vi "Decode_Int16.vi"(1 "Little Endian":u8[](array[numeric])) -> (0 "Int16":i16[](array[numeric]))   [LabVIEW 2015, in "navX Library v3.lvlib" / "navX Registry Cache.lvclass"]
uses:
  navX Registry Cache.lvclass
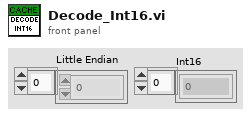
[diagram p1: front panel]
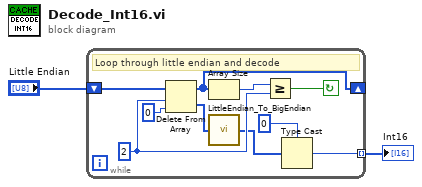
[diagram p0: block diagram]
diagram:
  n1 = while {
    shift-right: [w3] -> _
    shift-left: "Little Endian" -> [w7]
    tunnel: [w5] -> w1 mode=indexing
    stop <- w4 continue-if-true
    w9 = 2 ("length")
    # "Loop through little endian and decode"
    n2 = Delete From Array(array=w7, length=w9, index=0) -> (deleted portion=w8:u8[], array with subset deleted=w3:u8[])
    n3 = Array Size(array=w3) -> (size(s)=w10:i32)
    n4 = call "LittleEndian_To_BigEndian.vi"("Little Endian"=w8) -> ("Big Endian"=w6:u8[])
    n5 = Greater Or Equal?(x=w10, y=w9) -> (x >= y?=w4:bool)
    n6 = Type Cast(type=i16 0, x=w6) -> (*(type *) &x=w5:i16)
  }
  "Int16" <- w1
